vi "addslashes.vi"(11 "input string":string="\\\\192.168.1.5\\data\\EN\\1. UPDATE\\KIEM KE") -> (3 "addslashes":string)   [LabVIEW 2015]
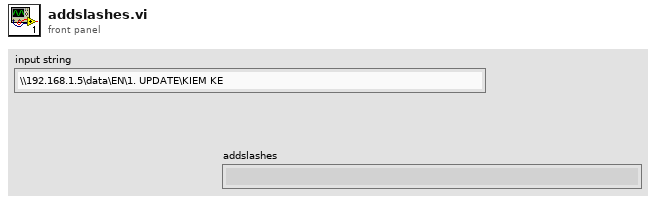
[diagram p1: front panel]
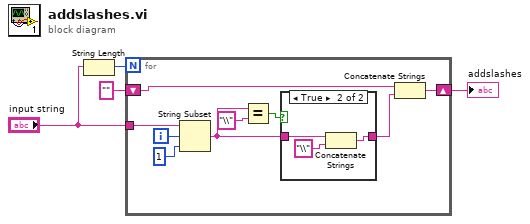
[diagram p0: block diagram]
diagram:
  n1 = String Length(string="input string") -> (length=w3:i32)
  n2 = for {
    N: w3 -> [_]
    shift-right: [w11] -> w4
    shift-left: "" -> [w6]
    tunnel: "input string" -> [w5]
    i -> [w9]
    n3 = String Subset(string=w5, offset (0)=w9, length (rest)=1 ("length (rest)")) -> (substring=w7:string)
    n4 = Equal?(x=w7, y="\\") -> (x = y?=w12:bool)
    n5 = case shown="True" w12 {
      tunnel: [w14 w16] -> w10
      tunnel: w7 -> [w14 w15]
      frame False {
      }
      frame True {
        n6 = Concatenate Strings(w15, "\\" ("string")) -> (w16:string)
      }
    }
    n7 = Concatenate Strings(w6, w10) -> (w11:string)
  }
  "addslashes" <- w4
